vi "ConfigLCR.vi"(0 "VISA resource name LCR":refnum<visa-resource-name>, 11 "error in (no error)":errorcluster) -> (4 "VISA resource name out":refnum<visa-resource-name>, 15 "error out":errorcluster)   [LabVIEW 2015]
uses:
  Program Files (x86)/National Instruments/LabVIEW 2016/instr.lib/Agilent 428X Series/Agilent 428X Series.lvlib
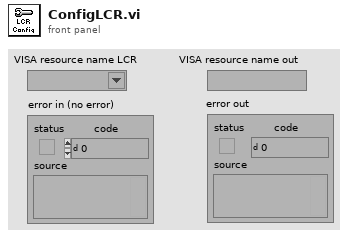
[diagram p1: front panel]
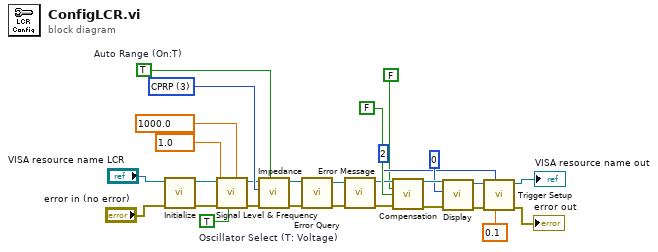
[diagram p0: block diagram]
diagram:
  w10 = u32 3 items=["CPD", "CPQ", "CPG", "CPRP", "CSD", "CSQ", "CSRS", "LPQ", "LPD", "LPG", "LPRP", "LSD", "LSQ", "LSRS", "RX", "ZTD", "ZTR", "GB", "YTD", "YTR"] ("Imp Type (0: CPD)")
  w11 = TRUE  # Oscillator Select (T: Voltage)
  w7 = TRUE  # Auto Range (On:T)
  n1 = call "Initialize.vi"("error in (no error)"="error in (no error)", "VISA resource name"="VISA resource name LCR") -> ("error out"=w19:errorcluster, "VISA resource name out"=w18:refnum<visa-resource-name>)  [unwired: 8 in]
  n2 = call "Signal Level & Frequency.vi"("Frequency Value (Hz) (100KHz)"=1000.0 ("Freq Value (Hz)(1.0 kHz)"), "Oscillator Select (T: Voltage)"=w11, "error in (no error)"=w19, "Voltage Level (V) (5mV)"=1.0 ("Voltage Level (V)(1.0V)"), "VISA resource name"=w18) -> ("error out"=w6:errorcluster, "VISA resource name out"=w5:refnum<visa-resource-name>)  [unwired: 5 in]
  n3 = call "Impedance.vi"("Auto Range (F: Off)"=w7, "error in (no error)"=w6, "Imp Type (0: CPD)"=w10, "VISA resource name"=w5) -> ("error out"=w12:errorcluster, "VISA resource name out"=w13:refnum<visa-resource-name>)  [unwired: 6 in]
  n4 = call "Error Query.vi"("error in (no error)"=w12, "VISA resource name"=w13) -> ("error out"=w20:errorcluster, "VISA resource name out"=w14:refnum<visa-resource-name>)  [unwired: 6 in, 2 out]
  n5 = call "Error Message.vi"("error in (no error)"=w20, "VISA resource name"=w14) -> ("error out"=w15:errorcluster, "VISA resource name out"=w16:refnum<visa-resource-name>)  [unwired: 5 in, 3 out]
  n6 = call "Compensation.VI"("VISA resource name"=w16, "OPEN (F:OFF)"=FALSE ("Open (F:OFF)"), "SHORT (F:OFF)"=FALSE ("Short (F:OFF)"), "error in (no error)"=w15) -> ("VISA resource name out"=w27:refnum<visa-resource-name>, "error out"=w26:errorcluster)  [unwired: 10 in]
  n7 = call "Display.vi"("error in (no error)"=w26, "Display Page (0: Measurement)"=u32 0 ("Display Page (Measurment:0)"), "VISA resource name"=w27) -> ("error out"=w24:errorcluster, "VISA resource name out"=w25:refnum<visa-resource-name>)  [unwired: 7 in]
  n8 = call "Trigger Setup.vi"("Delay Value (s) (0.0)"=0.1, "Trigger Source (0: Internal)"=u32 2 ("bus triggering"), "error in (no error)"=w24, "VISA resource name"=w25) -> ("error out"=→"error out":errorcluster, "VISA resource name out"=→"VISA resource name out":refnum<visa-resource-name>)  [unwired: 6 in]
